vi "mod_MSK Transmitter.vi"(0 "Symbol Rate, Hz":dbl=1.0 format="%.2f", 1 "Reset?":bool=TRUE, 2 "# Samples per Symbol":i32=16, 5 "Differential Encoding":enum16{"disable", "enable"}(ring)=enum."enable", 7 "Message":T2={"# Guard Bits"=2, "# Sync Bits"=20, "# Message Bits"=1000, "PN sequence order"=9}, 9 "System Filter":T1={"TX Filter"=enum."Gaussian", "BT"=0.5, "filter length"=8} {"BT" format="%.2f"}, 11 "error in (no error)":errorcluster) -> (4 "Output Complex Waveform":T4 {"Y" format="%.3f"; "dt" format="%^.2e"; "t0" format="%.4f"}, 6 "Signal Description":T3={"Output Bit Stream"=[], " # bits per symbol"=0, "Sync (Bits)"=[], "Sync (Symbols)"=[], "pulse shaping filter coefficients"=[], "matched filter coefficients"=[], "MSK system parameters"={"differential encoding enable"=enum."enable", "samples per symbol (16)"=16}} {"matched filter coefficients" format="%.2f"; "pulse shaping filter coefficients" format="%.2f"; "Sync (Symbols)" format="%.2f"}, 15 "error out":errorcluster)   [LabVIEW 2020, in "niDMT.lvlib"]
doc: "This example demonstrates gneration of a MSK modulated signal. You can specify characteristics of the message signal such as PN sequence order, number of guard bits, number of sync bits, and transmit filter parameters. You can extend this example to download the generated MSK signal to GPIB-based RF signal generators."
uses:
  <vilib>/addons/Modulation/niDMT.lvlib
  <vilib>/addons/Modulation/Analog/controls/Complex Data Waveform.ctl
  <vilib>/addons/Modulation/Analog/support/mod_Set Error Source.vi
  <vilib>/addons/Modulation/Digital/Support/Common/Validators/mod_Generate Filter Coefficients Validate.vi
  <vilib>/addons/Modulation/Digital/General/subVIs/mod_Generate Filter Coefficients.vi
  <vilib>/addons/Modulation/Digital/General/MT Generate MSK System Parameters.vi
  <vilib>/addons/Modulation/niAMT.lvlib
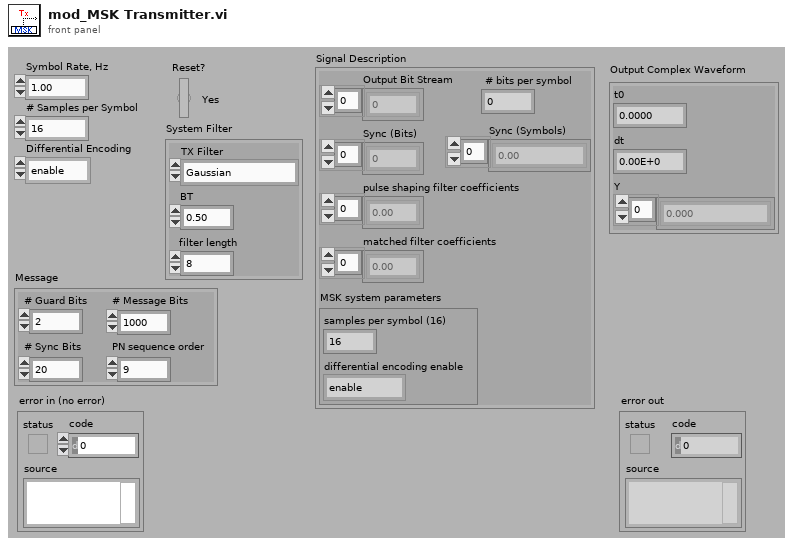
[diagram p1: front panel]
types:
  T1 = cluster{"TX Filter":enum16{"none", "Raised Cosine", "Root Raised Cos", "Gaussian"}, "BT":dbl, "filter length":i32}
  T2 = cluster{"# Guard Bits":i32, "# Sync Bits":i32, "# Message Bits":i32, "PN sequence order":i32}
  T3 = cluster{"Output Bit Stream":i8[], " # bits per symbol":i32, "Sync (Bits)":i8[], "Sync (Symbols)":cdb[], "pulse shaping filter coefficients":dbl[], "matched filter coefficients":dbl[], "MSK system parameters":cluster{"differential encoding enable":enum16{"disable", "enable"}, "samples per symbol (16)":i32}}
  T4 = typedef "niAMT.lvlib/Complex Data Waveform.ctl" = cluster{"t0":dbl, "dt":dbl, "Y":cdb[]}
  T5 = cluster{"Output Bit Stream":i8[], "# bits per symbol":i32, "Sync (Bits)":i8[], "Sync (Symbols)":cdb[], "pulse shaping filter coefficients":dbl[], "matched filter coefficients":dbl[], "MSK system parameters":cluster{"differential encoding enable":enum16{"disable", "enable"}, "samples per symbol (16)":i32}}
  T6 = enum16{"none", "Raised Cosine", "Root Raised Cos", "Gaussian"}
  T7 = cluster{"differential encoding enable":enum16{"disable", "enable"}, "samples per symbol (16)":i32}
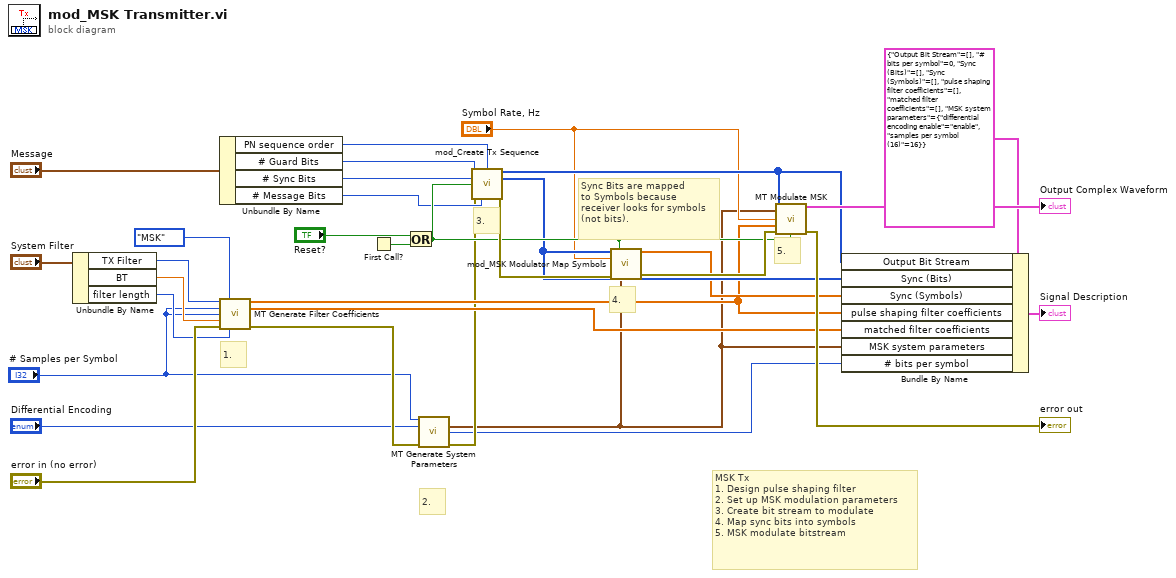
[diagram p0: block diagram]
diagram:
  # "5."
  # "4."
  # "2."
  # "3."
  # "1."
  # "MSK Tx\n1. Design pulse shaping filter\n2. Set up MSK modulation parameters\n3. Create bit stream to modulate\n4. Map sync bits into symbols\n5. MSK modulate bitstream"
  # "Sync Bits are mapped\nto Symbols because\nreceiver looks for symbols\n(not bits)."
  n1 = Unbundle By Name("System Filter") -> ("TX Filter"=w19:T6, "BT"=w18:dbl, "filter length"=w17:i32)
  n2 = Unbundle By Name("Message") -> ("PN sequence order"=w11:i32, "# Guard Bits"=w23:i32, "# Sync Bits"=w22:i32, "# Message Bits"=w21:i32)
  n3 = call <vilib>:"MT Generate Filter Coefficients.vi"("pulse shaping filter (none)"=w19, "modulation type"=enum16{"FSK", "PSK", "QAM", "MSK", "PAM", "ASK"}."MSK", "pulse shaping samples per symbol (16)"="# Samples per Symbol", "matched samples per symbol (16)"="# Samples per Symbol", "filter parameter"=w18, "error in (no error)"="error in (no error)", "filter length (symbols)"=w17) -> ("pulse shaping filter coefficients"=w13:dbl[], "matched filter coefficients"=w12:dbl[], "error out"=w7:errorcluster)  [unwired: 6 out]
  n4 = First Call?() -> (First Call?: T/F=w27:bool)
  n5 = Or(x="Reset?", y=w27) -> (x .or. y?=w25:bool)
  n6 = call-poly <vilib>:"MT Generate System Parameters.vi"("samples per symbol (16)"="# Samples per Symbol", "differential encoding enable"="Differential Encoding", "error in (no error)"=w7) -> ("MSK system parameters"=w2:T7, "bits per symbol"=w3:i32, "error out"=w4:errorcluster)  [unwired: 10 out]
  n7 = call <vilib>:"mod_Create Tx Sequence.vi"("# Guard Bits (2)"=w23, "PN sequence order (9)"=w11, "# Sync Bits (20)"=w22, "Reset? (T)"=w25, "error in (no error)"=w4, "# Message Bits"=w21) -> ("Output Bit Stream"=w16:i8[], "Last Sync Pattern"=w15:i8[], "error out"=w30:errorcluster)  [unwired: 3 in, 4 out]
  n8 = call <vilib>:"mod_MSK Modulator Map Symbols.vi"("Input Bit Stream"=w15, "MSK System Parameters"=w2, "Symbol Rate, Hz"="Symbol Rate, Hz", "error in (no error)"=w30, "Reset? (T)"=w25) -> ("Symbols Out"=w14:dbl[], "error out"=w31:errorcluster)  [unwired: 1 in, 8 out]
  n9 = call <vilib>:"MT Modulate MSK.vi"("input bit stream"=w16, "MSK system parameters"=w2, "symbol rate (Hz)"="Symbol Rate, Hz", "pulse shaping filter coefficients"=w13, "error in (no error)"=w31, "reset? (T)"=w25) -> ("output complex waveform"=→"Output Complex Waveform":T4, "error out"=→"error out":errorcluster)  [unwired: 1 in, 7 out]
  n10 = Bundle By Name(cluster=T5 {"Output Bit Stream"=[], "# bits per symbol"=0, "Sync (Bits)"=[], "Sync (Symbols)"=[], "pulse shaping filter coefficients"=[], "matched filter coefficients"=[], "MSK system parameters"={"differential encoding enable"=enum."enable", "samples per symbol (16)"=16}} ("Signal Description"), "Output Bit Stream"=w16, "Sync (Bits)"=w15, "Sync (Symbols)"=w14, "pulse shaping filter coefficients"=w13, "matched filter coefficients"=w12, "MSK system parameters"=w2, "# bits per symbol"=w3) -> (→"Signal Description":T5)
